vi "Write Control.vi"(8 "error in (no error)":errorcluster, 10 "Control":u16, 11 "Storage Line in":refnum<class "Storage Line.lvclass">) -> (0 "error out":errorcluster, 3 "Storage Line out":refnum<class "Storage Line.lvclass">)   [LabVIEW 2015, in "cRIO-Carbondioxide.lvlib" / "CO2-Actor.lvlib" / "Storage Line.lvclass"]
uses:
  Storage Line.lvclass
  Storage Line.lvclass/Storage Line.ctl
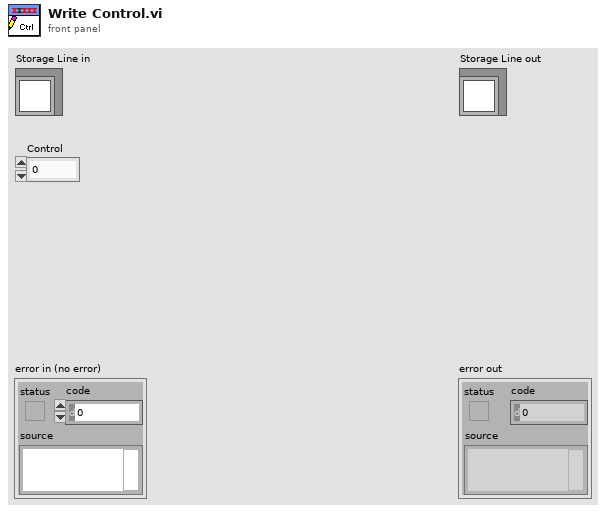
[diagram p1: front panel]
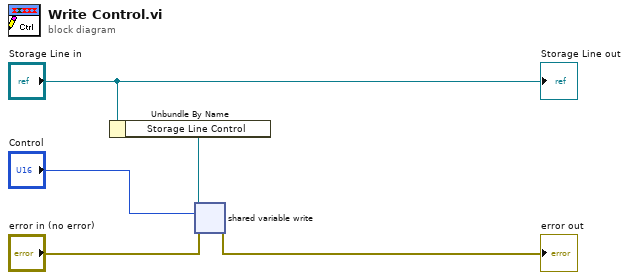
[diagram p0: block diagram]
diagram:
  n1 = Unbundle By Name("Storage Line in") -> ("Storage Line Control"=w2:refnum<k21>)
  n2 = shared-variable-write(w2, "error in (no error)", "Control") -> (→"error out":errorcluster)  [unwired: 1 out]
  "Storage Line out" <- "Storage Line in"
